vi "matlabDOwffromparam.vi"(1 "waveform params":T1) -> (0 "digital waveform":digitalwaveform(waveform))   [LabVIEW 2015]
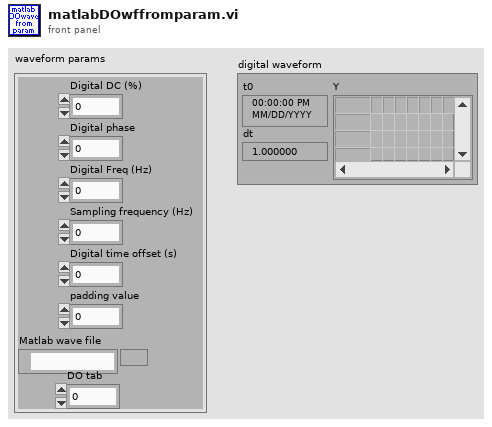
[diagram p1: front panel]
types:
  T1 = cluster{"Digital DC (%)":dbl, "Digital phase":dbl, "Digital Freq (Hz)":dbl, "Sampling frequency (Hz)":dbl, "Digital time offset (s) ":dbl, "padding value":dbl, "Matlab wave file":path, "DO tab":dbl}
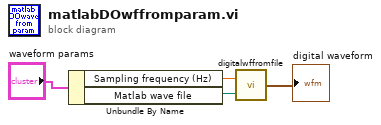
[diagram p0: block diagram]
diagram:
  n1 = Unbundle By Name("waveform params") -> ("Sampling frequency (Hz)"=w1:dbl, "Matlab wave file"=w2:path)
  n2 = call "digitalwffromfile.vi"("Matlab wave file"=w2, "Sampling frequency (Hz)"=w1) -> ("digital waveform"=→"digital waveform":digitalwaveform)
